vi "Inserisci codice.vi"() -> (0 "TIPO out":string, 1 "Modalità out":T1(ring), 2 "ANNULLA":bool, 3 "Codice out":string)   [LabVIEW 2019]
panel:
  in  "TIPO":string(combo)
  in  "Modalità":T1(radio)
  out "x = y?":bool
  in  "ANNULLA":bool
  in  "CONFERMA CODICE":bool
  in  "CODICE":string
  # "INSERISCI IL CODICE COLLAUDO"
  # ">>"
  # "<<"
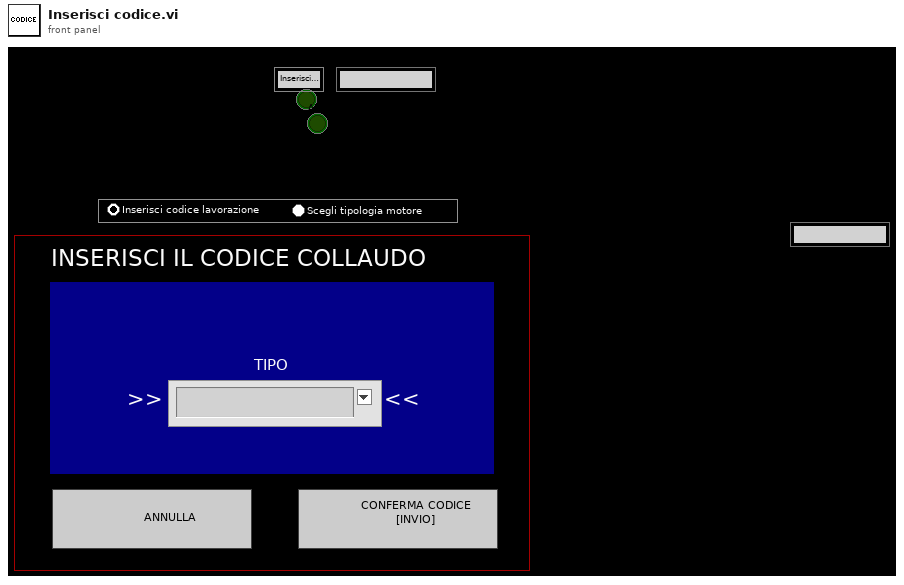
[diagram p1: front panel]
types:
  T1 = enum32{"Inserisci codice lavorazione", "Scegli tipologia motore"}
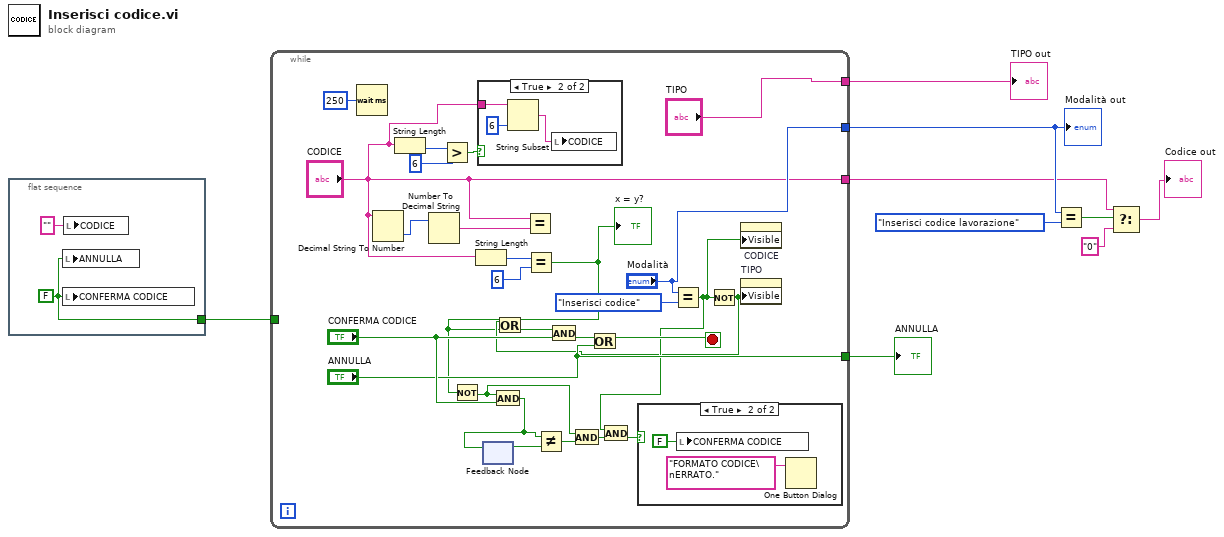
[diagram p0: block diagram]
diagram:
  n1 = flat-sequence {
    tunnel: [w10] -> w8
    frame #0 {
      w10 = FALSE ("CONFERMA CODICE")
      n2 = local write "ANNULLA"(w10) -> ()
      n3 = local write "CONFERMA CODICE"(w10) -> ()
      n4 = local write "CODICE"("" ("CODICE")) -> ()
    }
  }
  n5 = while {
    tunnel: ["CODICE"] -> w3
    tunnel: ["ANNULLA"] -> w9
    tunnel: w8 -> [_]
    tunnel: ["Modalità"] -> w6
    tunnel: ["TIPO"] -> w7
    stop <- w27 stop-if-true
    n6 = Wait (ms)(milliseconds to wait=u32 250) -> ()  [unwired: 1 out]
    n7 = Decimal String To Number(string="CODICE") -> (number=w37:i32)  [unwired: 2 in, 1 out]
    n8 = String Length(string="CODICE") -> (length=w30:i32)
    n9 = Number To Decimal String(number=w37) -> (decimal integer string=w35:string)  [unwired: 1 in]
    n10 = Greater?(x=w30, y=6) -> (0:w28:bool)
    n11 = String Length(string="CODICE") -> (length=w34:i32)
    n12 = case shown="True" w28 {
      tunnel: "CODICE" -> [_ w40]
      frame False {
      }
      frame True {
        n13 = String Subset(string=w40, length (rest)=6 ("length (rest)")) -> (substring=w38:string)  [unwired: 1 in]
        n14 = local write "CODICE"(w38) -> ()
      }
    }
    n15 = feedback #1() -> (w24:bool)  [unwired: 1 in]
    n16 = Equal?(x="CODICE", y=w35) -> ()  [unwired: 1 out]
    n17 = Equal?(x=w34, y=6) -> (x = y?=w13:bool)
    "x = y?" <- w13
    n18 = Not(x=w13) -> (.not. x?=w21:bool)
    n19 = And(x=w21, y="CONFERMA CODICE") -> (x .and. y?=w25:bool)
    n20 = feedback-in #1(w25) -> ()
    n21 = Not Equal?(x=w25, y=w24) -> (x != y?=w23:bool)
    n22 = And(x=w21, y=w23) -> (x .and. y?=w22:bool)
    n23 = Equal?(x="Modalità", y=enum32{"Inserisci codice", "Scegli manualmente"}."Inserisci codice") -> (x = y?=w16:bool)
    n24 = And(x=w16, y=w22) -> (x .and. y?=w17:bool)
    n25 = case shown="True" w17 {
      frame False {
      }
      frame True {
        n26 = local write "CONFERMA CODICE"(FALSE ("CONFERMA CODICE")) -> ()
        n27 = One Button Dialog(message="FORMATO CODICE\nERRATO.") -> ()  [unwired: 1 in, 1 out]
      }
    }
    n28 = Not(x=w16) -> (.not. x?=w14:bool)
    n29 = Or(x=w14, y=w13) -> (x .or. y?=w15:bool)
    n30 = And(x=w15, y="CONFERMA CODICE") -> (x .and. y?=w32:bool)
    n31 = Or(x=w32, y="ANNULLA") -> (x .or. y?=w27:bool)
    n32 = property on="CODICE" class="Str"("Visible"=w16) -> ()  [unwired: 2 in, 2 out]
    n33 = property on="TIPO" class="CmbBox"("Visible"=w14) -> ()  [unwired: 2 in, 2 out]
  }
  "ANNULLA" <- w9
  "Modalità out" <- w6
  "TIPO out" <- w7
  n34 = Equal?(x=w6, y=T1."Inserisci codice lavorazione") -> (x = y?=w5:bool)
  n35 = Select(t=w3, s=w5, f="0") -> (s? t:f=→"Codice out":string)
